vi "Execute New VI From Template.vi"(6 "Mouse Position":T2, 8 "User VI Ref":refnum<vi>, 9 "Menu Item Tag Suffix":string, 10 "Remaining Items":refnum<vi>[](array[refnum]), 11 "Affected Items":cluster{"Any Refnums":refnum<vi>[]}) -> (0 "Fail transaction?":bool)   [LabVIEW 2021]
doc: "This VI is part of a plug-in for modifying the LabVIEW shortcut menus. This is the execute VI which is called when the shortcut menu is chosen by the user. It performs the action of the selected menu item."
uses:
  <vilib>/Utility/miscctls.llb/LVPositionTypeDef.ctl
  Owner Status.ctl
  GUI Objects.ctl
  Testing Flag (enum).ctl
  Testing Flag (library variable).vi
panel:
  in  "SCL":i32(listbox) caption="Templates"
  in  "OK Button":bool
  in  "Apply Owner Icon Template?":bool
  out "error out":errorcluster
  out "Owner Filename (including extension)":string
  out "User VI Owner Status":T1
  out "Owner Path":path
  out "Iteration":i32
  out "Tab":enum32{"SomeTemplatesFound", "NoTemplatesFound"}(tab)
  in  "Create":bool
  in  "Destination Location":path
  in  "Add To Owner?":bool caption="Add to Library 1.lvlib?"
  in  "Add To Project?":bool caption="Add to Project?"
  in  "Open Front Panel?":bool caption="Open Front Panel When Created?"
  in  "Project ComboBox":string(combo) caption="Project"
  out "NoTemplatesFound Message":string
  # "Execute VI"
  # "Not user-facing"
  # "All controls on this panel except \"Affected Items\" have been locked to prevent accidental edits. Changing the control names or types, other than the elements of the \"Affected Items\" cluster will make the VI unusable as a menu plugin.\n\nSee Context Help for each control for details about its use."
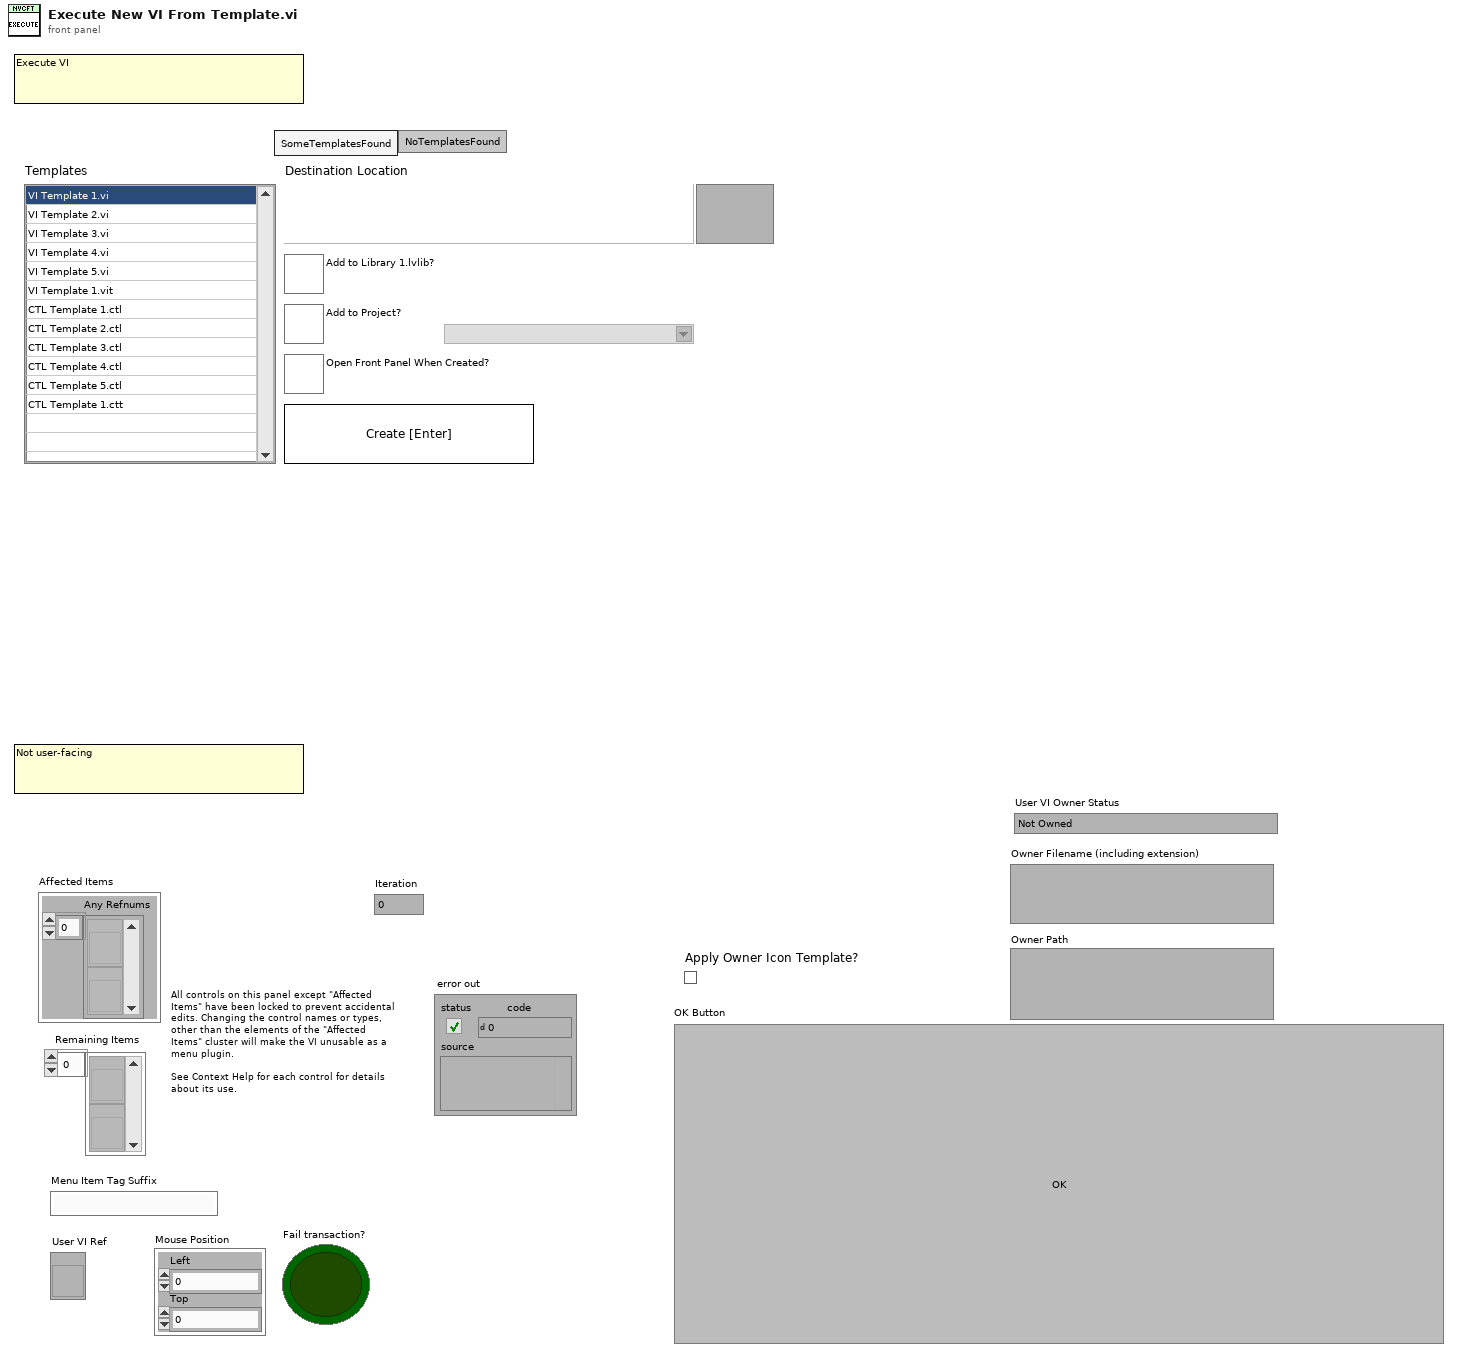
[diagram p1: front panel]
types:
  T1 = typedef "Owner Status.ctl" = enum16{"Not Owned", "Owned by Library (lvlib)", "Owned by Class (lvclass)"}
  T2 = typedef "LVPositionTypeDef.ctl" = cluster{"Left":i32, "Top":i32}
  T3 = typedef "GUI Objects.ctl" = cluster{"SCL":refnum<vi>, "Add To Owner?":refnum<vi>, "Add To Project?":refnum<vi>, "Open Front Panel?":refnum<vi>, "Destination Folder":refnum<vi>, "Create":refnum<vi>, "Project ComboBox":refnum<vi>, "NoTemplatesFound Message":refnum<vi>}
  T4 = typedef "Testing Flag (enum).ctl" = enum16{"Production", "Testing"}
  T5 = enum32{"Invalid", "Standard", "Closed", "Hidden", "Minimized", "Maximized"}
  T6 = enum8{"Enabled", "Disabled", "Disabled and Grayed Out"}
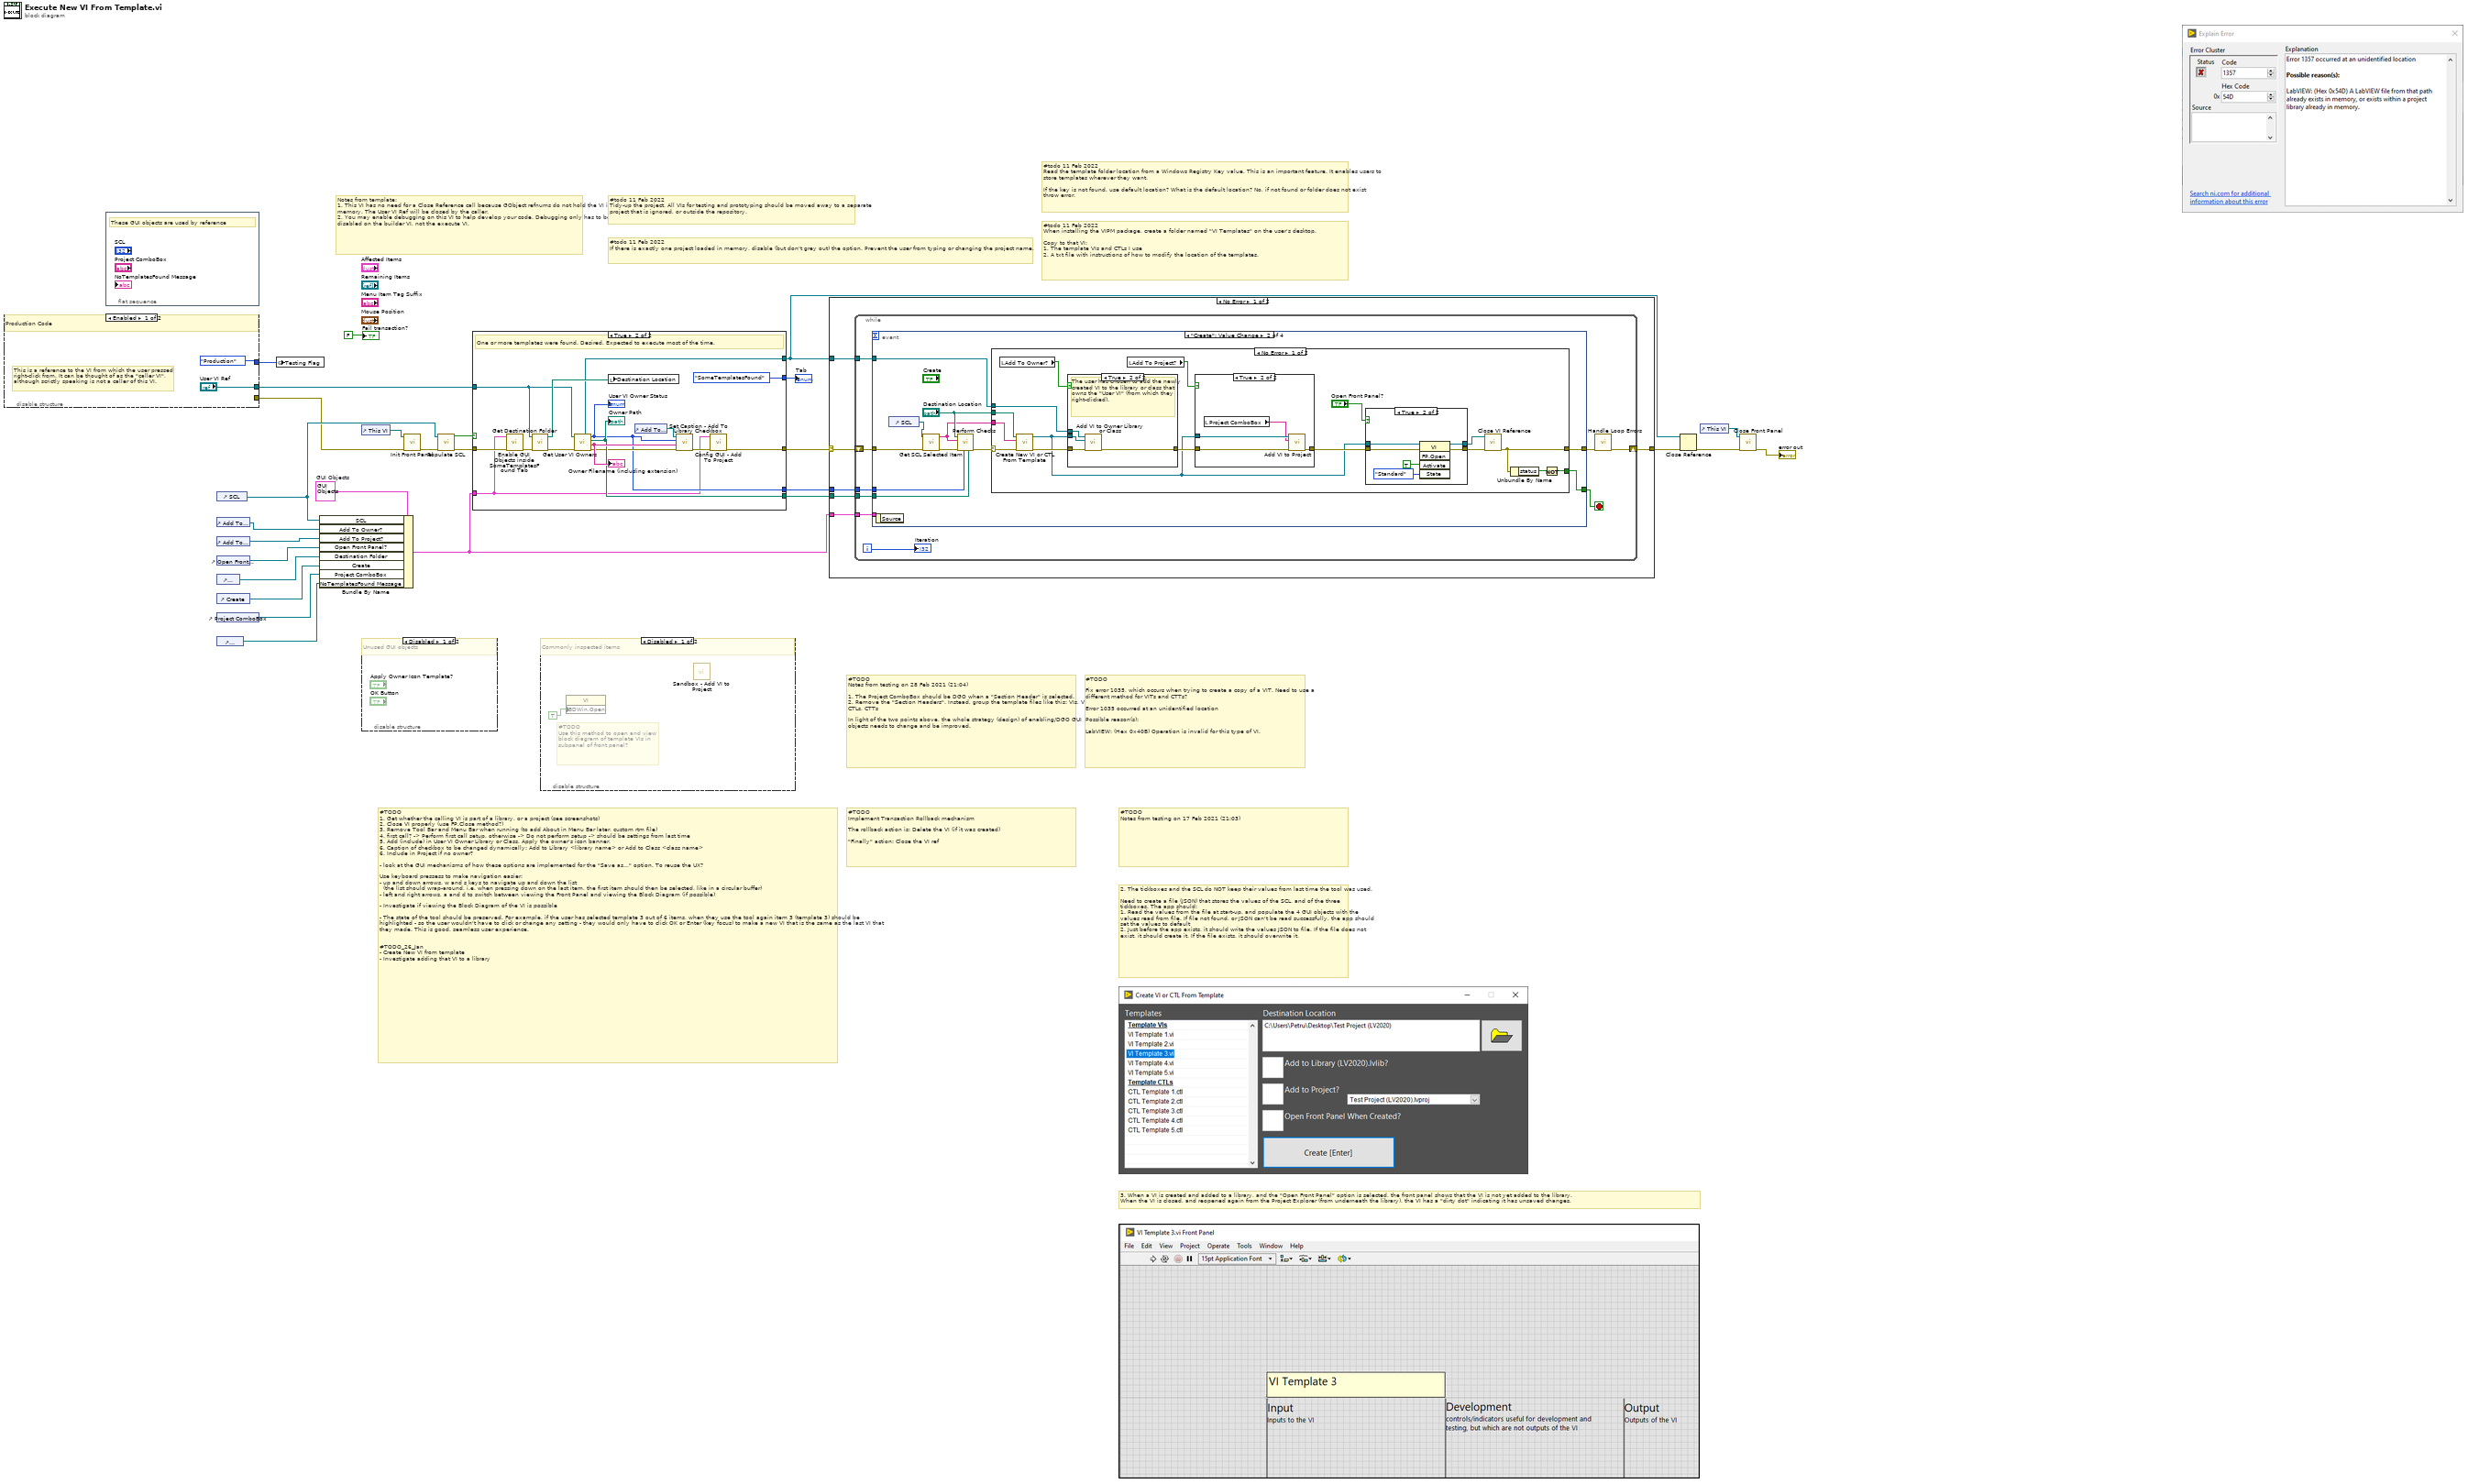
[diagram p0: block diagram]
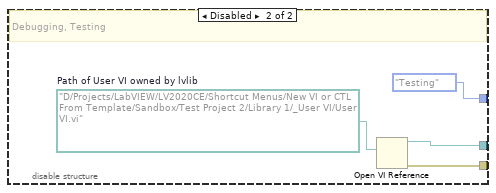
[diagram p3: hidden frame]
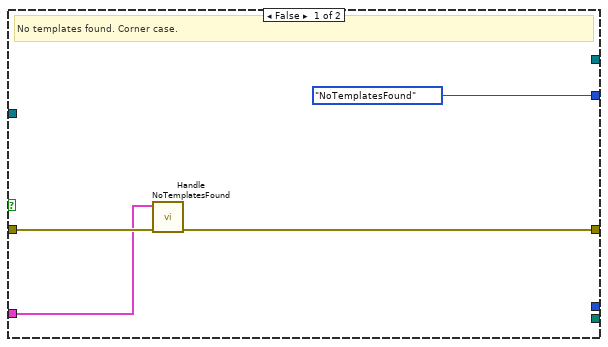
[diagram p4: hidden frame]
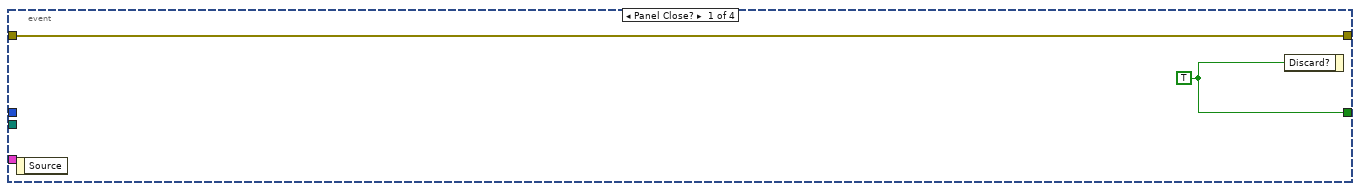
[diagram p6: hidden frame]
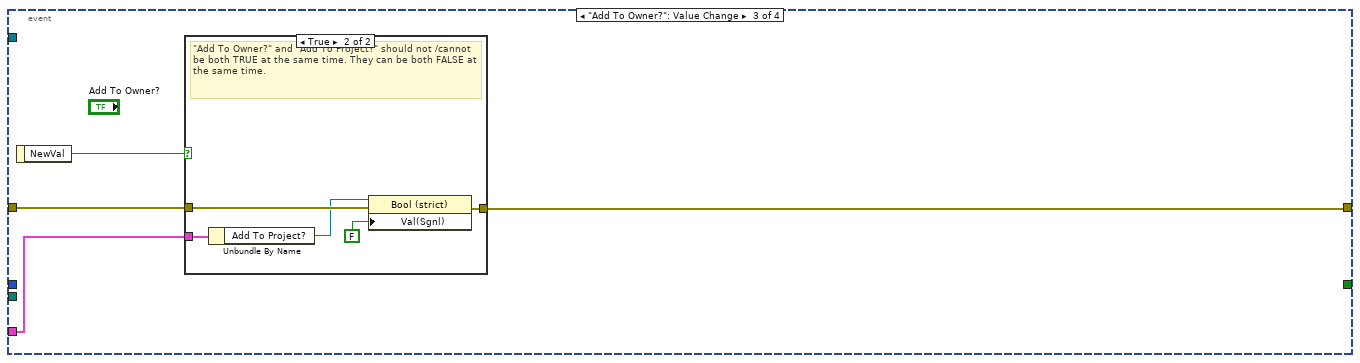
[diagram p11: hidden frame]
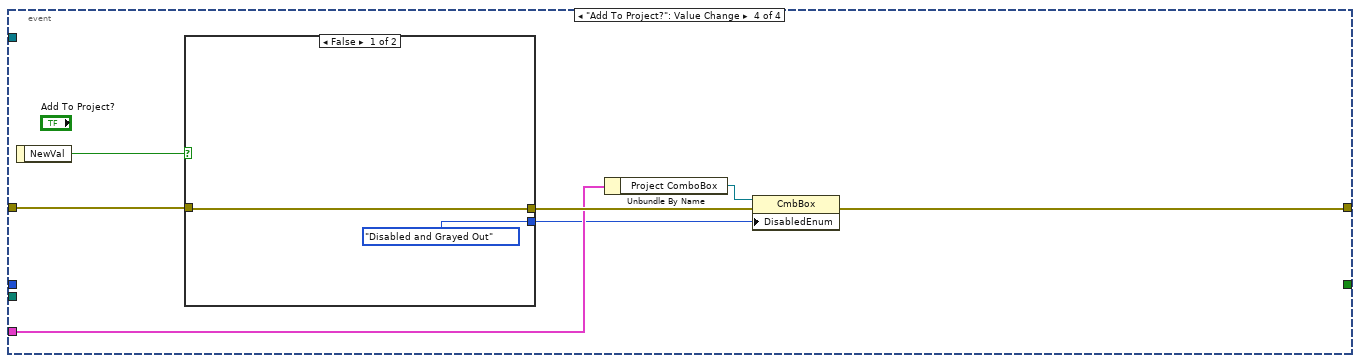
[diagram p13: hidden frame]
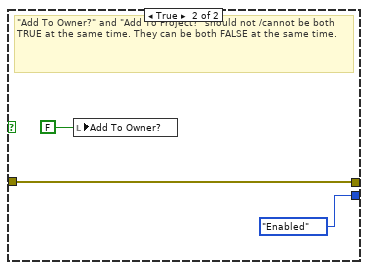
[diagram p14: hidden frame]
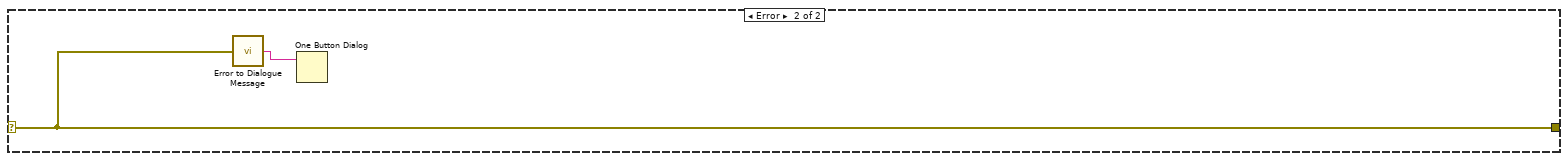
[diagram p15: hidden frame]
diagram:
  w20 = T3 {"SCL"=refnum, "Add To Owner?"=refnum, "Add To Project?"=refnum, "Open Front Panel?"=refnum, "Destination Folder"=refnum, "Create"=refnum, "Project ComboBox"=refnum, "NoTemplatesFound Message"=refnum}  # GUI Objects
  # "#todo 11 Feb 2022\nWhen installing the VIPM package, create a folder named \"VI Templates\" on the user's desktop.\n\nCopy to that VI:\n1. The template VIs and CTLs I use\n2. A txt file with instructions of how to modify the location of the templates."
  # "#todo 11 Feb 2022\nRead the template folder location from a Windows Registry Key value. This is an important feature. It enables users to store templates wherever they want.\n\nIf the key is not found, use default location? What is the default location? No, if not found or folder does not exist throw error."
  # "#todo 11 Feb 2022\nTidy-up the project. All VIs for testing and prototyping should be moved away to a separate project that is ignored, or outside the repository."
  # "#todo 11 Feb 2022\nIf there is exactly one project loaded in memory, disable (but don't grey out) the option. Prevent the user from typing or changing the project name."
  # "#TODO\nNotes from testing on 28 Feb 2021 (21:04)\n\n1. The Project ComboBox should be DGO when a \"Section Header\" is selected.\n2. Remove the \"Section Headers\". Instead, group the template files like this: VIs, VITs, CTLs, CTTs\n\nIn light of the two points above, the whole strategy (design) of enabling/DGO GUI objects needs to change and be improved."
  # "#TODO\n\nFix error 1035, which occurs when trying to create a copy of a VIT. Need to use a different method for VITs and CTTs?\n\nError 1035 occurred at an unidentified location\n\nPossible reason(s):\n\nLabVIEW: (Hex 0x40B) Operation is invalid for this type of VI."
  # "2. The tickboxes and the SCL do NOT keep their values from last time the tool was used.\n\nNeed to create a file (JSON) that stores the values of the SCL, and of the three tickboxes. The app should:\n1. Read the values from the file at start-up, and populate the 4 GUI objects with the values read from file. If file not found, or JSON can't be read successfully, the app should set the values to default\n2. Just before the app exists, it should write the values JSON to file. If the file does not exist, it should create it. If the file exists, it should overwrite it."
  # "3. When a VI is created and added to a library, and the \"Open Front Panel\" option is selected, the front panel shows that the VI is not yet added to the library.\nWhen the VI is closed, and reopened again from the Project Explorer (from underneath the library), the VI has a \"dirty dot\" indicating it has unsaved changes."
  # "#TODO\nNotes from testing on 17 Feb 2021 (21:03)"
  # "#TODO\nImplement Transaction Rollback mechanism\n\nThe rollback action is: Delete the VI (if it was created)\n\n\"Finally\" action: Close the VI ref"
  # "#TODO\n1. Get whether the calling VI is part of a library, or a project (see screenshots)\n2. Close VI properly (use FP.Close method?)\n3. Remove Tool Bar and Menu Bar when running (to add About in Menu Bar later, custom rtm file)\n4. first call? -> Perform first call setup. otherwise -> Do not perform setup -> should be settings from last time\n5. Add (include) in User VI Owner Library or Class. Apply the owner's icon banner.\n6. Caption of checkbox to be changed dynamically: Add to Library <library name> or Add to Class <class name>\n6. Include in Project if no owner?\n\n- look at the GUI mechanisms of how these options are implemented for the \"Save as...\" option. To reuse the UX?\n\nUse keyboard pressess to make navigation easier:\n- up and down arrows, w and s keys to navigate up and down the list\n  (the list should wrap-around, i.e. when pressing down on the last item, the first item should then be selected, like in a circular buffer)\n- left and right arrows, a and d to switch between viewing the Front Panel and viewing the Block Diagram (if possible)\n\n- Investigate if viewing the Block Diagram of the VI is possible\n\n- The state of the tool should be preserved. For example, if the user has selected template 3 out of 6 items, when they use the tool again item 3 (template 3) should be highlighted - so the user wouldn't have to click or change any setting - they would only have to click OK or Enter (key focus) to make a new VI that is the same as the last VI that they made. This is good, seamless user experience.\n\n\n#TODO_26_Jan\n- Create New VI from template\n- Investigate adding that VI to a library"
  # "Notes from template:\n1. This VI has no need for a Close Reference call because GObject refnums do not hold the VI in memory. The User VI Ref will be closed by the caller.\n2. You may enable debugging on this VI to help develop your code. Debugging only has to be disabled on the builder VI, not the execute VI."
  n1 = disable-structure shown="Enabled" {
    disable-tunnel: ["User VI Ref" w31] -> w15
    disable-tunnel: [Testing_Flag_(enum)."Production" ("Testing Flag") Testing_Flag_(enum)."Testing" ("Testing Flag")] -> w10
    disable-tunnel: [_ w30] -> w7
    frame Enabled {
      # "This is a reference to the VI from which the user pressed right-click from. It can be thought of as the \"caller VI\", although scrictly speaking is not a caller of this VI."
      # "Production Code"
    }
    frame Disabled {
      w32 = path "D:/Projects/LabVIEW/LV2020CE/Shortcut Menus/New VI or CTL From Template/Sandbox/Test Project 2/Library 1/_User VI/User VI.vi"  # Path of User VI owned by lvlib
      # "Debugging, Testing"
      n2 = Open VI Reference(vi path=w32) -> (vi reference=w31:refnum<vi>, error out=w30:errorcluster)  [unwired: 5 in]
    }
  }
  n3 = flat-sequence {
    frame #0 {
      # "These GUI objects are used by reference"
    }
  }
  n4 = control-ref of="SCL"() -> (w19:refnum<vi>)
  n5 = control-ref of="Add To Owner?"() -> (w18:refnum<vi>)
  n6 = control-ref of="Add To Project?"() -> (w14:refnum<vi>)
  n7 = control-ref of="Open Front Panel?"() -> (w13:refnum<vi>)
  n8 = control-ref of="Destination Location"() -> (w17:refnum<vi>)
  n9 = control-ref of="Create"() -> (w16:refnum<vi>)
  n10 = control-ref of="Project ComboBox"() -> (w6:refnum<vi>)
  n11 = control-ref of="NoTemplatesFound Message"() -> (w1:refnum<vi>)
  n12 = global write "Testing Flag (library variable).vi" "Testing Flag"(w10) -> ()
  n13 = Bundle By Name(cluster=w20, "SCL"=w19, "Add To Owner?"=w18, "Add To Project?"=w14, "Open Front Panel?"=w13, "Destination Folder"=w17, "Create"=w16, "Project ComboBox"=w6, "NoTemplatesFound Message"=w1) -> (w4:T3)
  n14 = control-ref of="This VI"() -> (w26:refnum<vi>)
  n15 = disable-structure shown="Disabled" {
    frame Disabled {
      # "Unused GUI objects"
    }
    frame Enabled {
    }
  }
  n16 = call "Init Front Panel.vi"("error in"=w7, "VI Reference"=w26) -> ("error out"=w25:errorcluster)  [unwired: 9 in]
  n17 = call "Populate SCL.vi"("error in"=w25, "SCL"=w19) -> ("error out"=w12:errorcluster, "At least one template file found?"=w3:bool)  [unwired: 8 in]
  n18 = case shown="True" w3 {
    tunnel: [_ w47] -> w21
    tunnel: w15 -> [_ w46]
    tunnel: w12 -> [w37 w44]
    tunnel: [_ w43] -> w11
    tunnel: [_ w42] -> w8
    tunnel: [w35 w41] -> w5
    tunnel: w4 -> [w34 w38]
    tunnel: [enum32{"SomeTemplatesFound", "NoTemplatesFound"}."NoTemplatesFound" ("Tab") enum32{"SomeTemplatesFound", "NoTemplatesFound"}."SomeTemplatesFound" ("Tab")] -> w2
    frame False {
      # "No templates found. Corner case."
      n19 = call "Handle NoTemplatesFound.vi"("error in"=w37, "GUI Objects"=w34) -> ("error out"=w35:errorcluster)  [unwired: 9 in]
    }
    frame True {
      # "One or more templates were found. Desired. Expected to execute most of the time."
      n20 = call "Enable GUI Objects inside SomeTemplatesFound Tab.vi"("error in"=w44, "GUI Objects"=w38) -> ("error out"=w39:errorcluster)  [unwired: 9 in]
      n21 = call "Get Destination Folder.vi"("error in"=w39, "User VI Ref"=w46) -> ("error out"=w52:errorcluster, "Destination Folder"=w48:path)  [unwired: 8 in]
      n22 = call "Get User VI Owners.vi"("error in"=w52, "User VI Ref"=w46) -> ("error out"=w45:errorcluster, "Owner Filename (inc file extension)"=w49:string, "Owner Path"=w47:path, "User VI Owner Status"=w43:T1, "Owner Reference"=w42:refnum<vi>)  [unwired: 4 in, 1 out]
      "Owner Path" <- w47
      "User VI Owner Status" <- w43
      "Owner Filename (including extension)" <- w49
      n23 = local write "Destination Location"(w48) -> ()
      n24 = control-ref of="Add To Owner?"() -> (w50:refnum<vi>)
      n25 = call "Set Caption - Add To Library Checkbox.vi"("error in"=w45, "Owner Filename (including extension)"=w49, "User VI Owner Status"=w43, "Add To Owner"=w50) -> ("error out"=w51:errorcluster)  [unwired: 7 in]
      n26 = call "Config GUI - Add To Project.vi"("error in"=w51, "GUI Objects"=w38) -> ("error out"=w41:errorcluster)  [unwired: 8 in, 1 out]
    }
  }
  "Tab" <- w2
  n27 = disable-structure shown="Disabled" {
    frame Disabled {
      # "#TODO\nUse this method to open and view block diagram of template VIs in subpanel of front panel?"
      # "Commonly inspected items"
      n28 = property class="VI"("BDWin.Open"=TRUE ("Block Diagram Window:Open")) -> ()  [unwired: 2 in, 2 out]
      n29 = call "Sandbox - Add VI to Project.vi"() -> ()  [unwired: 11 in, 1 out]
    }
    frame Enabled {
    }
  }
  n30 = case shown="No Error" w5 {
    selector: w5 -> [w59 w140]
    tunnel: [w58 w140] -> w24
    tunnel: w11 -> [w57 _]
    tunnel: w21 -> [w56 _]
    tunnel: w4 -> [w55 _]
    tunnel: w8 -> [w54 _]
    frame No Error {
      n31 = while {
        shift-right: [w62] -> w58
        shift-left: w59 -> [w68]
        tunnel: w57 -> [w65]
        tunnel: w56 -> [w64]
        tunnel: w55 -> [w61]
        tunnel: w54 -> [w60]
        i -> [w67]
        stop <- w66 stop-if-true
        n32 = event shown="[1] \"Create\": Value Change" {
          selector: _ -> [_ _ _ _]
          dyn-events: _ -> [_ _ _ _]
          timeout: _ -> [_ _ _ _]
          tunnel: w68 -> [w69 w80 w119 w132]
          tunnel: [w70 w72 _ _] -> w66
          tunnel: [w69 w81 w118 w130] -> w63
          tunnel: w65 -> [_ w77 _ _]
          tunnel: w64 -> [_ w76 _ _]
          tunnel: w61 -> [_ _ w117 w129]
          tunnel: w60 -> [_ w73 _ _]
          event Panel Close? {
            w70 = TRUE
            n33 = event-data() -> ()  [unwired: 1 in, 1 out]
            n34 = event-data("Discard?"=w70) -> ()  [unwired: 1 in, 1 out]
          }
          event "Create": Value Change {
            n35 = event-data() -> ()  [unwired: 1 in, 1 out]
            n36 = control-ref of="SCL"() -> (w71:refnum<vi>)
            n37 = call "Get SCL Selected Item.vi"("error in"=w80, "SCL"=w71) -> ("error out"=w79:errorcluster, "Selected Item (String)"=w74:string)  [unwired: 7 in, 1 out]
            n38 = call "Perform Checks.vi"("Owner Path (if applicable)"=w76, "User VI Owner Status"=w77, "error in"=w79, "Selected Template VI or CTL name (including file extension)"=w74, "Destination Folder"="Destination Location") -> ("error out"=w78:errorcluster)  [unwired: 6 in]
            n39 = case shown="No Error" w78 {
              selector: w78 -> [w97 w116]
              tunnel: [w84 w116] -> w81
              tunnel: "Destination Location" -> [w96 _]
              tunnel: w74 -> [w95 _]
              tunnel: w73 -> [w92 _]
              tunnel: [w82 _] -> w72
              frame No Error {
                n40 = local read "Add To Owner?"() -> (w94:bool)
                n41 = call "Create New VI or CTL From Template.vi"("error in"=w97, "Selected Template VI or CTL name (including file extension)"=w95, "Destination Folder"=w96) -> ("error out"=w93:errorcluster, "Reference of newly created VI"=w85:refnum<vi>)  [unwired: 7 in]
                n42 = case shown="True" w94 {
                  tunnel: [w103 w107] -> w88
                  tunnel: w93 -> [w103 w106]
                  tunnel: w85 -> [_ w105]
                  tunnel: w92 -> [_ w104]
                  frame False {
                  }
                  frame True {
                    # "The user has chosen to add the newly created VI to the library or class that owns the \"User VI\" (from which they right-clicked)."
                    n43 = call "Add VI to Owner Library or Class.vi"("error in"=w106, "Reference of newly created VI"=w105, "Owner Reference (Library or Class)"=w104) -> ("error out"=w107:errorcluster)  [unwired: 8 in]
                  }
                }
                n44 = local read "Add To Project?"() -> (w86:bool)
                n45 = case shown="True" w86 {
                  tunnel: [w98 w102] -> w87
                  tunnel: w88 -> [w98 w101]
                  tunnel: w85 -> [_ w100]
                  frame False {
                  }
                  frame True {
                    n46 = local read "Project ComboBox"() -> (w99:string)
                    n47 = call "Add VI to Project.vi"("error in"=w101, "Add VI to this Project"=w99, "Reference of newly created VI or CTL"=w100) -> ("error out"=w102:errorcluster)  [unwired: 8 in]
                  }
                }
                n48 = case shown="True" "Open Front Panel?" {
                  tunnel: w87 -> [w109 w115]
                  tunnel: [w109 w114] -> w91
                  tunnel: w85 -> [w108 w113]
                  tunnel: [w108 w110] -> w90
                  frame False {
                  }
                  frame True {
                    n49 = invoke class="VI" method="FP.Open"(reference=w113, error in=w115, "Activate"=TRUE ("Activate?"), "State"=T5."Standard") -> (reference out=w110:refnum<vi>, error out=w114:errorcluster)  [unwired: 1 in, 3 out]
                  }
                }
                n50 = call "Close VI Reference.vi"("error in"=w91, "VI Reference"=w90) -> ("error out"=w84:errorcluster)  [unwired: 9 in]
                n51 = Unbundle By Name(w84) -> ("status"=w83:bool)
                n52 = Not(x=w83) -> (.not. x?=w82:bool)
              }
              frame Error {
              }
            }
          }
          event "Add To Owner?": Value Change {
            n53 = event-data() -> ("NewVal"=w120:bool)  [unwired: 1 in]
            n54 = case shown="True" w120 {
              tunnel: w119 -> [w121 w126]
              tunnel: [w121 w125] -> w118
              tunnel: w117 -> [_ w124]
              frame False {
              }
              frame True {
                # "\"Add To Owner?\" and \"Add To Project?\" should not /cannot be both TRUE at the same time. They can be both FALSE at the same time."
                n55 = Unbundle By Name(w124) -> ("Add To Project?"=w123:refnum<vi>)
                n56 = property class="Bool (strict)"(reference=w123, error in=w126, "Val(Sgnl)"=FALSE ("Value (Signaling)")) -> (error out=w125:errorcluster)  [unwired: 1 out]
              }
            }
          }
          event "Add To Project?": Value Change {
            n57 = event-data() -> ("NewVal"=w133:bool)  [unwired: 1 in]
            n58 = case shown="False" w133 {
              tunnel: w132 -> [w135 w137]
              tunnel: [w135 w137] -> w131
              tunnel: [T6."Disabled and Grayed Out" ("Disabled") T6."Enabled" ("Disabled")] -> w127
              frame False {
              }
              frame True {
                # "\"Add To Owner?\" and \"Add To Project?\" should not /cannot be both TRUE at the same time. They can be both FALSE at the same time."
                n59 = local write "Add To Owner?"(FALSE ("Add To Project?")) -> ()
              }
            }
            n60 = Unbundle By Name(w129) -> ("Project ComboBox"=w128:refnum<vi>)
            n61 = property class="CmbBox"(reference=w128, error in=w131, "DisabledEnum"=w127) -> (error out=w130:errorcluster)  [unwired: 1 out]
          }
        }
        n62 = call "Handle Loop Errors.vi"("error in"=w63) -> ("error out"=w62:errorcluster)  [unwired: 10 in]
        "Iteration" <- w67
      }
    }
    frame Error {
      n63 = call "Error to Dialogue Message.vi"("error in"=w140) -> ("Dialogue Message"=w139:string)
      n64 = One Button Dialog(message=w139) -> ()  [unwired: 1 in, 1 out]
    }
  }
  n65 = Close Reference(reference=w8, error in (no error)=w24) -> (error out=w9:errorcluster)
  n66 = control-ref of="This VI"() -> (w23:refnum<vi>)
  n67 = call "Close Front Panel.vi"("error in"=w9, "VI Reference"=w23) -> ("error out"=→"error out":errorcluster)  [unwired: 9 in]
  "Fail transaction?" <- FALSE ("Fail transaction?")
